vi "Send Message.vi"(8 "error in (no error)":errorcluster, 10 "Message":string, 11 "Serial Communication in":refnum<class "Serial Communication.lvclass">) -> (0 "error out":errorcluster, 3 "Serial Communication out":refnum<class "Serial Communication.lvclass">)   [LabVIEW 2018, in "Serial Communication.lvclass"]
uses:
  Serial Communication.lvclass
  Serial Communication.lvclass/Serial Communication.ctl
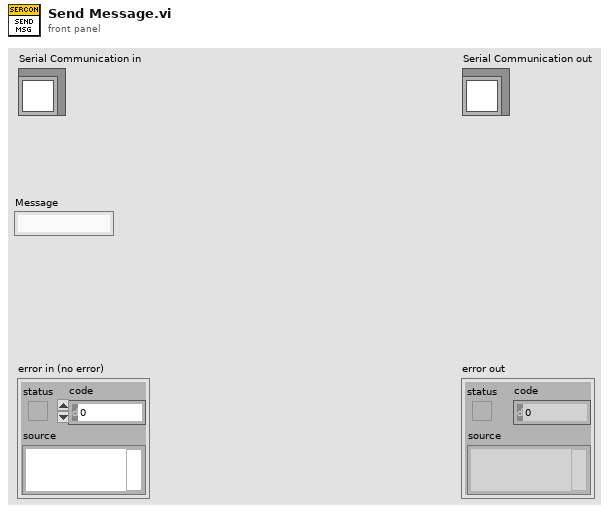
[diagram p1: front panel]
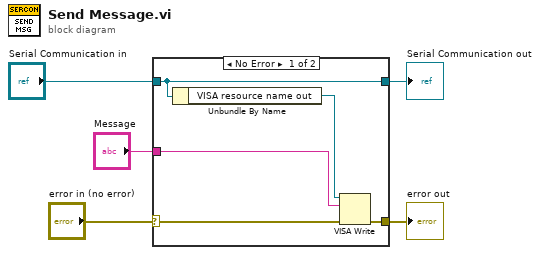
[diagram p0: block diagram]
diagram:
  n1 = case shown="No Error" "error in (no error)" {
    selector: "error in (no error)" -> [w8 w12]
    tunnel: [w7 w12] -> w2
    tunnel: [w10 w11] -> w3
    tunnel: "Serial Communication in" -> [w10 w11]
    tunnel: "Message" -> [w6 _]
    frame No Error {
      n2 = Unbundle By Name(w10) -> ("VISA resource name out"=w9:refnum<visa-resource-name>)
      n3 = VISA Write(VISA resource name=w9, write buffer=w6, error in (no error)=w8) -> (error out=w7:errorcluster)  [unwired: 2 out]
    }
    frame Error {
    }
  }
  "error out" <- w2
  "Serial Communication out" <- w3
